vi "broadcaster.vi"(4 "port":u16, 6 "timeout":u32, 7 "Subnet Local Broadcast Address in":string, 9 "enable":bool, 10 "read buffer":string, 11 "use 255.255.255.255(true) or subnet local broadcast ip(false)?":bool) -> (0 "error out":errorcluster, 3 "Current Broadcast Address out":string)   [LabVIEW 2017]
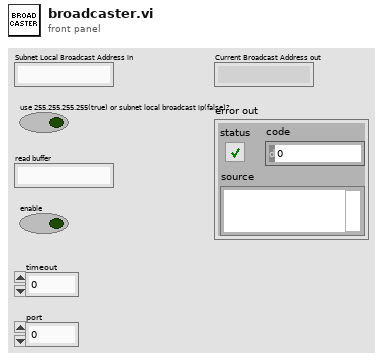
[diagram p1: front panel]
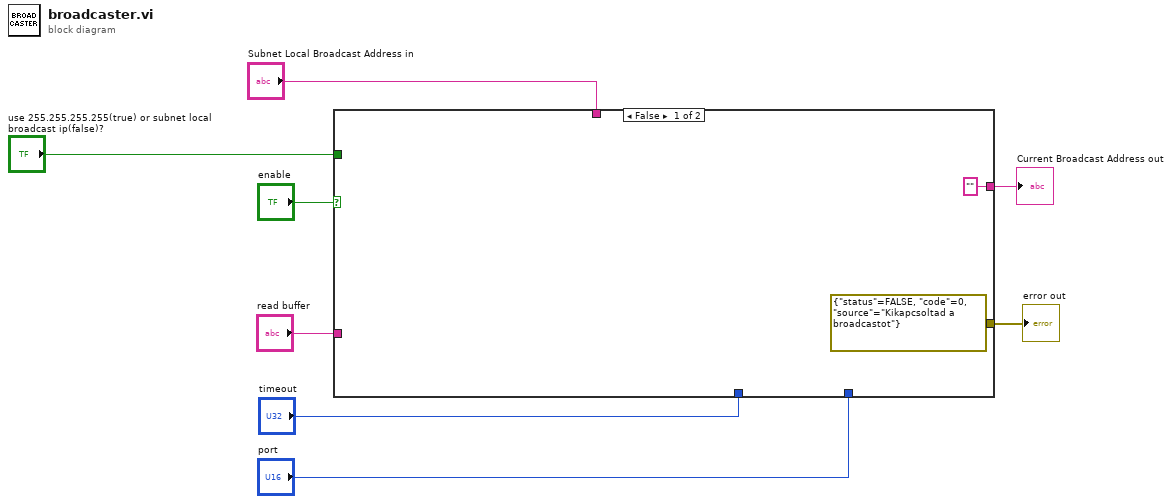
[diagram p0: block diagram]
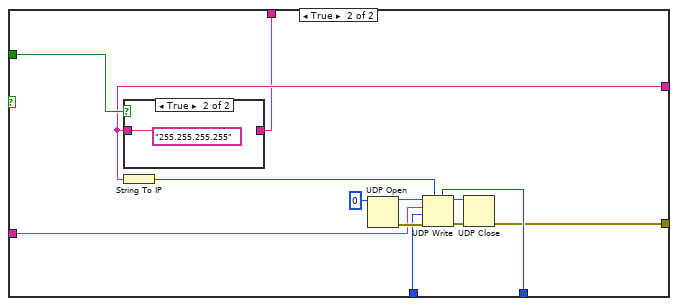
[diagram p2: hidden frame]
diagram:
  n1 = case shown="False" "enable" {
    tunnel: "timeout" -> [_ w20]
    tunnel: "read buffer" -> [_ w14]
    tunnel: "port" -> [_ w19]
    tunnel: "use 255.255.255.255(true) or subnet local broadcast ip(false)?" -> [_ w17]
    tunnel: ["" ("Subnet Local Broadcast Address") w16] -> w6
    tunnel: "Subnet Local Broadcast Address in" -> [_ w15]
    tunnel: [errorcluster {"status"=FALSE, "code"=0, "source"="Kikapcsoltad a broadcastot"} ("error out") w11] -> w8
    frame False {
    }
    frame True {
      n2 = case shown="True" w17 {
        tunnel: w15 -> [w24 _]
        tunnel: [w24 "255.255.255.255"] -> w16
        frame False {
        }
        frame True {
        }
      }
      n3 = String To IP(1:w16) -> (0:w18:u32)
      n4 = UDP Open(11:u16 0 ("port")) -> (port=w22:refnum<k16>, 0:w23:errorcluster)  [unwired: 4 in, 1 out]
      n5 = UDP Write(address=w18, port or service name=w19, connection ID=w22, data in=w14, 8:w23, 9:w20) -> (error out=w13:errorcluster, 3:w12:refnum<k16>)
      n6 = UDP Close(connection ID=w12, 8:w13) -> (error out=w11:errorcluster)  [unwired: 1 out]
    }
  }
  "error out" <- w8
  "Current Broadcast Address out" <- w6
